vi "SetUIState.vi"(8 "error in (no error)":errorcluster, 10 "UI State":T1=enum."Embedded", 11 "EmbeddedSMO in":refnum<class "SMO.UI.Embedded.lvclass">) -> (0 "error out":errorcluster, 3 "EmbeddedSMO out":refnum<class "SMO.UI.Embedded.lvclass">)   [LabVIEW 2020, in "SMO.UI.Embedded.lvclass"]
uses:
  SMO.UI.Embedded.lvclass
  Typedefs/UI State.ctl
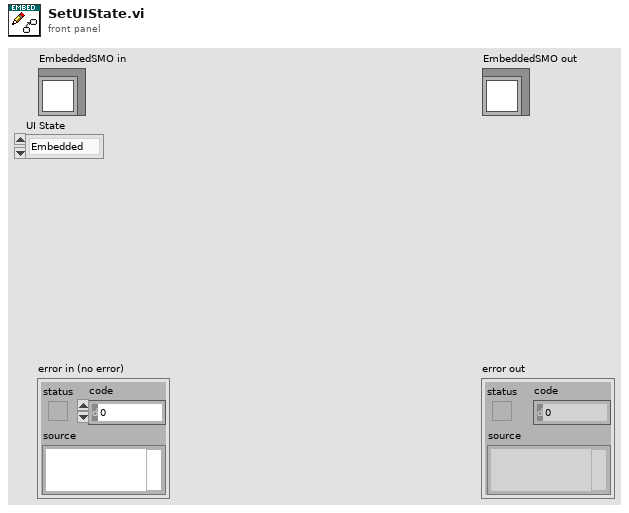
[diagram p1: front panel]
types:
  T1 = typedef "SMO.UI.Embedded.lvclass/UI State.ctl" = enum16{"unknown", "Opened", "Embedded", "Closed"}
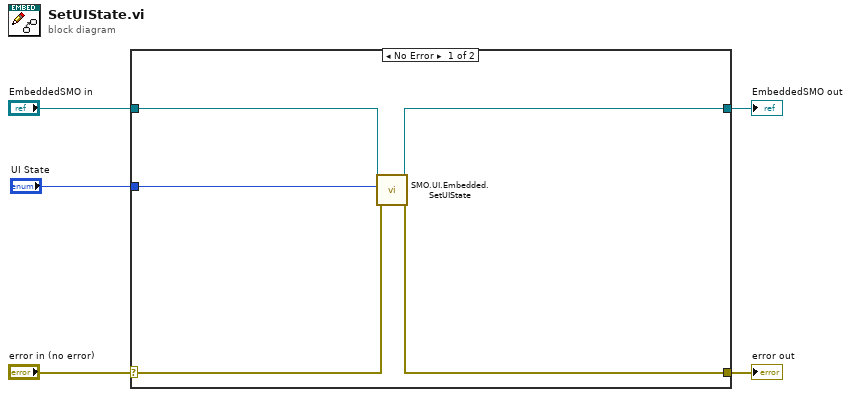
[diagram p0: block diagram]
diagram:
  n1 = case shown="No Error" "error in (no error)" {
    selector: "error in (no error)" -> [w7 w12]
    tunnel: [w6 w12] -> w4
    tunnel: [w9 w11] -> w2
    tunnel: "EmbeddedSMO in" -> [w10 w11]
    tunnel: "UI State" -> [w8 _]
    frame No Error {
      n2 = call "SMO.UI.Embedded.SetUIState.vi"("error in (no error)"=w7, "UI State"=w8, "EmbeddedSMO"=w10) -> ("error out"=w6:errorcluster, "EmbeddedSMO out"=w9:refnum<class "SMO.UI.Embedded.lvclass">)  [unwired: 7 in]
    }
    frame Error {
    }
  }
  "error out" <- w4
  "EmbeddedSMO out" <- w2
